vi "ReadConfigTemp.vi"(2 "Error In":errorcluster, 3 "Configs":string) -> (0 "Error Out":errorcluster, 1 "tempTable":cluster{"ConfigTemps":T1[]})   [LabVIEW 2012]
uses:
  TempConfig.ctl
  <vilib>/LVH/i3 JSON/i3-json.lvlib
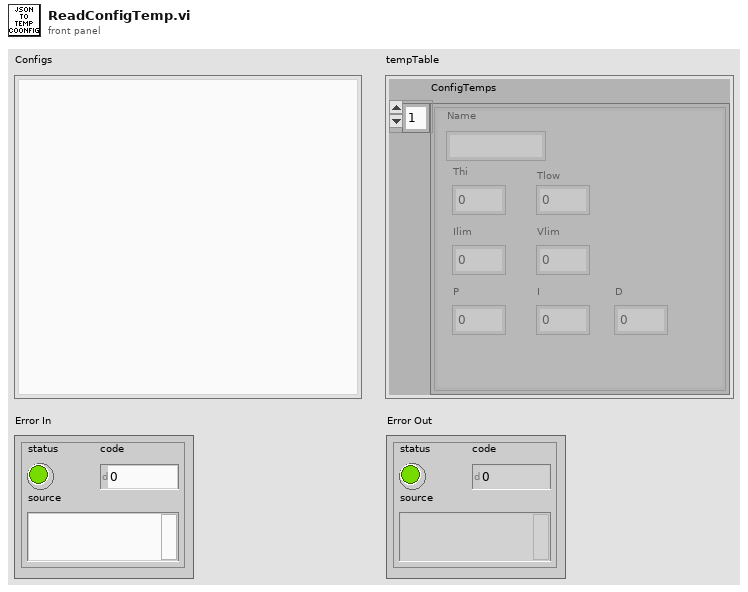
[diagram p1: front panel]
types:
  T1 = typedef "TempConfig.ctl" = cluster{"Name":string, "Thi":dbl, "Ilim":dbl, "P":dbl, "Tlow":dbl, "Vlim":dbl, "I":dbl, "D":dbl}
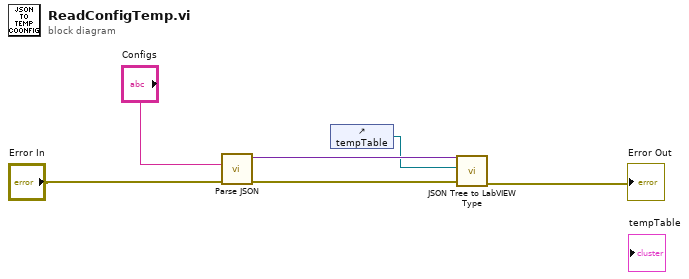
[diagram p0: block diagram]
diagram:
  n1 = call <vilib>:"Parse JSON.vi"("error in (no error)"="Error In", "JSON String"="Configs") -> ("error out"=w5:errorcluster, "JSON Tree"=w6:variant)  [unwired: 6 in, 2 out]
  n2 = control-ref of="tempTable"() -> (w3:refnum<vi>)
  n3 = call <vilib>:"JSON Tree to LabVIEW Type.vi"("error in (no error)"=w5, "Ctl Refnum"=w3, "JSON Tree In"=w6) -> ("error out"=→"Error Out":errorcluster)  [unwired: 7 in, 1 out]
